vi "Curl Height.vi"(0 "Image in":T1, 1 "Coord Centre X":dbl, 2 "Coord Centre Y":dbl, 3 "Angle":dbl, 4 "Overlay Enable":bool, 5 "Measurement ROI":T8={"Left"=40.0, "Top"=75.0, "Right"=80.0, "Bottom"=3.0, "Angle"=0.0}, 6 "Measu Edge Options":T5={"Edge Polarity"=0, "Kernel Size"=5, "Width"=5, "Minimum Edge Strength"=40.0, "Interpolation Type"=enum."Zero Order", "Data Processing Method"=enum."Average"} {"Edge Polarity" items=["All Edges", "Rising Edges", "Falling Edges"]; "Minimum Edge Strength" format="%.2f"; "Width" step=2; "Kernel Size" step=2}, 7 "error in (no error)":errorcluster, 8 "Measurement Reference ROI":T8={"Left"=0.0, "Top"=0.0, "Right"=0.0, "Bottom"=280.0, "Angle"=0.0}, 9 "Measu ROI Step Size":u32=1, 10 "Measu Ref Edge Options":T5={"Edge Polarity"=0, "Kernel Size"=5, "Width"=5, "Minimum Edge Strength"=40.0, "Interpolation Type"=enum."Zero Order", "Data Processing Method"=enum."Average"} {"Edge Polarity" items=["All Edges", "Rising Edges", "Falling Edges"]; "Minimum Edge Strength" format="%.2f"; "Width" step=2; "Kernel Size" step=2}, 11 "Measu ROI Process":T7(ring)=enum."Get First + Last Edge", 12 "Measu Ref Scan Direction":u16(ring)=2 items=["Left To Right", "Right To Left", "Top To Bottom", "Bottom To Top"], 13 "Measurement ROI Scan Direction":u16(ring) items=["Left To Right", "Right To Left", "Top To Bottom", "Bottom To Top"], 14 "Calibrated Image in":T1) -> (18 "Overlay Arrows Line":T2, 20 "Curl Height":dbl format="%.2f", 21 "min value":dbl, 22 "min index(es)":i32, 23 "Curl Min Point":cluster{"X":sgl, "Y":sgl}, 27 "error out":errorcluster)   [LabVIEW 2019, in "Algorithm.lvclass"]
uses:
  FrameworkOverrides/Algorithm.lvclass
  <vilib>/vision/NI_Vision_Development_Module.lvlib
  <vilib>/vision/Image Controls.llb/IMAQ Image.ctl
  <vilib>/vision/Measure.llb/Edge Polarity.ctl
  <vilib>/vision/Measure.llb/Edge Options.ctl
panel:
  out "Image out":T1(plugin-control)
  out "Second Overlay Line":T3
  out "First Overlay Line":T4
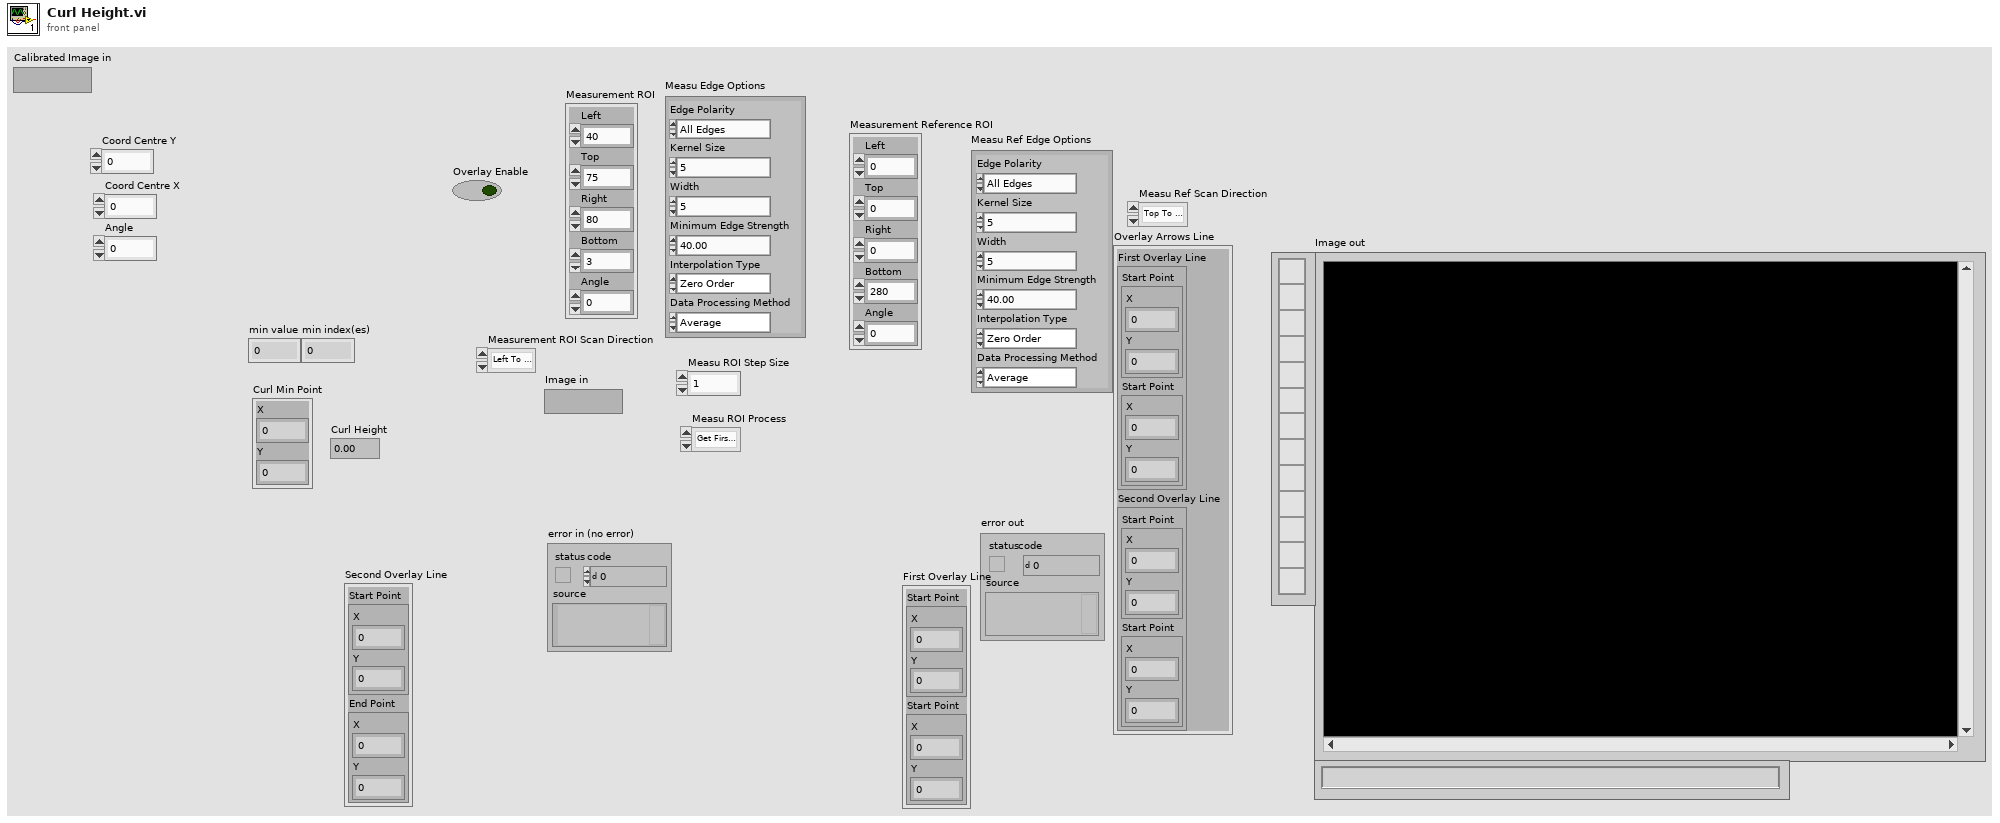
[diagram p1: front panel]
types:
  T1 = typedef "IMAQ Image.ctl" = refnum<image>
  T2 = cluster{"First Overlay Line ":cluster{"Start Point":cluster{"X":sgl, "Y":sgl}, "Start Point":cluster{"X":sgl, "Y":sgl}}, "Second Overlay Line ":cluster{"Start Point":cluster{"X":sgl, "Y":sgl}, "Start Point":cluster{"X":sgl, "Y":sgl}}}
  T3 = cluster{"Start Point":cluster{"X":sgl, "Y":sgl}, "End Point":cluster{"X":sgl, "Y":sgl}}
  T4 = cluster{"Start Point":cluster{"X":sgl, "Y":sgl}, "Start Point":cluster{"X":sgl, "Y":sgl}}
  T5 = typedef "Edge Options.ctl" = cluster{"Edge Polarity":T6, "Kernel Size":u32, "Width":u32, "Minimum Edge Strength":sgl, "Interpolation Type":enum32{"Zero Order", "Bilinear", "Quadratic", "Cubic", "Bilinear Fixed"}, "Data Processing Method":enum32{"Average", "Median"}}
  T6 = typedef "Edge Polarity.ctl" = u32
  T7 = enum16{"Get First Edge", "Get First + Last Edge", "Get All Edges", "Get Best Edge"}
  T8 = cluster{"Left":dbl, "Top":dbl, "Right":dbl, "Bottom":dbl, "Angle":dbl}
  T9 = typedef "Search Line.ctl" = cluster{"Start Point":cluster{"X":sgl, "Y":sgl}, "End Point":cluster{"X":sgl, "Y":sgl}, "Edge Info":T10[], "Edge Map":dbl[], "Calibration Valid":bool}
  T10 = typedef "Edge New.ctl" = cluster{"Location (Pixel)":cluster{"X":sgl, "Y":sgl}, "Location (Real-World)":cluster{"X":sgl, "Y":sgl}, "Distance (Pixel)":dbl, "Distance (Real-World)":dbl, "Strength":dbl, "Noise":dbl, "Rising?":bool}
  T11 = cluster{"Real World Coordinates":cluster{"X":sgl, "Y":sgl}, "Real World Coordinates":cluster{"X":sgl, "Y":sgl}}
  T12 = cluster{"Point 1":cluster{"X":sgl, "Y":sgl}, "Point 2":cluster{"X":sgl, "Y":sgl}}
  T13 = cluster{cluster{"X":sgl, sgl}, cluster{"X":sgl, "Y":sgl}}
  T14 = cluster{cluster{"X":sgl, "Y":sgl}, cluster{"X":sgl, sgl}}
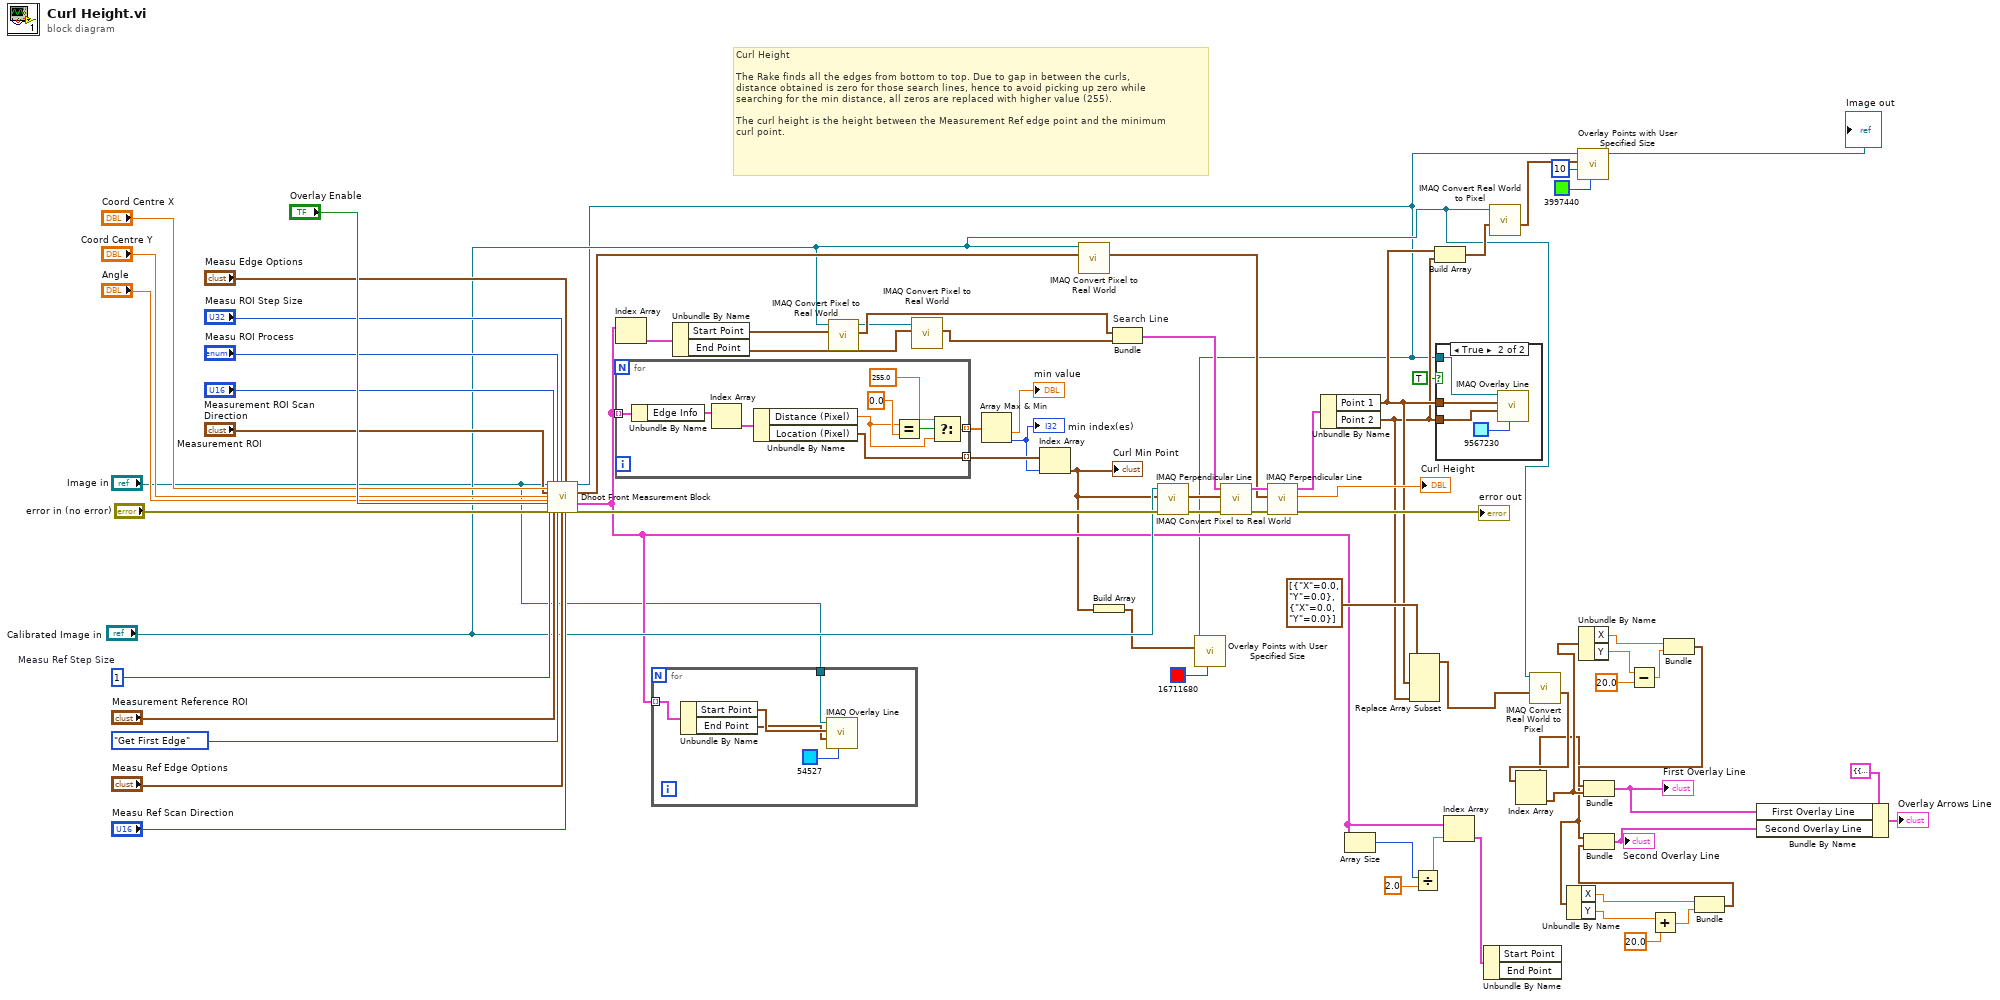
[diagram p0: block diagram]
diagram:
  w58 = u32 1  # Measu Ref Step Size
  # "Curl Height\n\nThe Rake finds all the edges from bottom to top. Due to gap in between the curls,\ndistance obtained is zero for those search lines, hence to avoid picking up zero while \nsearching for the min distance, all zeros are replaced with higher value (255).\n\nThe curl height is the height between the Measurement Ref edge point and the minimum \ncurl point."
  n1 = call "Dhoot Front Measurement Block.vi"("Image in"="Image in", "Coord Centre X"="Coord Centre X", "Measurement ROI"="Measurement ROI", "Coord Centre Y"="Coord Centre Y", "Angle"="Angle", "ROI Enable"="Overlay Enable", "Measu Ref Step Size"=w58, "error in (no error)"="error in (no error)", "Measurement ROI Scan Direction"="Measurement ROI Scan Direction", "Measurement Reference ROI"="Measurement Reference ROI", "Measu ROI Process"="Measu ROI Process", "Measu Ref Process"=T7."Get First Edge", "Measu ROI Step Size"="Measu ROI Step Size", "Measu Ref Edge Options"="Measu Ref Edge Options", "Measu Edge Options"="Measu Edge Options", "Measu Ref Scan Direction"="Measu Ref Scan Direction") -> ("Image out"=w2:T1, "Measu Ref Edge Point"=w39:cluster{"X":sgl, "Y":sgl}, "Search Lines"=w7:T9[], "error IO"=w47:errorcluster)  [unwired: 4 in, 4 out]
  "Image out" <- w2
  n2 = for {
    tunnel: w7 -> [w82] mode=indexing
    tunnel: [w75] -> w73 mode=indexing
    tunnel: [w74] -> w71 mode=indexing
    n3 = Unbundle By Name(w82) -> ("Edge Info"=w81:T10[])
    n4 = Index Array(array=w81) -> (element=w80:T10)  [unwired: 1 in]
    n5 = Unbundle By Name(w80) -> ("Distance (Pixel)"=w77:dbl, "Location (Pixel)"=w74:cluster{"X":sgl, "Y":sgl})
    n6 = Equal?(x=w77, y=0.0) -> (x = y?=w78:bool)
    n7 = Select(t=255.0, s=w78, f=w77) -> (s? t:f=w75:dbl)
  }
  n8 = Index Array(array=w7) -> (element=w69:T9)  [unwired: 1 in]
  n9 = for {
    tunnel: w7 -> [w87] mode=indexing
    tunnel: "Image in" -> [w84]
    n10 = Unbundle By Name(w87) -> ("Start Point"=w86:cluster{"X":sgl, "Y":sgl}, "End Point"=w85:cluster{"X":sgl, "Y":sgl})
    n11 = call "IMAQ Overlay Line"("Color"=u32 54527, "End Point"=w85, "Start Point"=w86, "Image"=w84) -> ()  [unwired: 6 in, 2 out]
  }
  n12 = Unbundle By Name(w69) -> ("Start Point"=w44:cluster{"X":sgl, "Y":sgl}, "End Point"=w42:cluster{"X":sgl, "Y":sgl})
  n13 = call "IMAQ Convert Pixel to Real World"("Pixel Coordinates"=w44, "Calibrated Image"="Calibrated Image in") -> ("Real World Coordinates"=w43:cluster{"X":sgl, "Y":sgl}, "Calibrated Image (duplicate)"=w40:T1)  [unwired: 4 in, 4 out]
  n14 = call "IMAQ Convert Pixel to Real World"("Pixel Coordinates"=w42, "Calibrated Image"=w40) -> ("Real World Coordinates"=w41:cluster{"X":sgl, "Y":sgl})  [unwired: 4 in, 5 out]
  n15 = Array Max & Min(array=w73) -> (min value=→"min value":dbl, min index (indices)=w70:i32)  [unwired: 2 out]
  "min index(es)" <- w70
  n16 = Index Array(array=w71, index=w70) -> (element=w4:cluster{"X":sgl, "Y":sgl})
  "Curl Min Point" <- w4
  n17 = call "IMAQ Convert Pixel to Real World"("Pixel Coordinates"=w39, "Calibrated Image"="Calibrated Image in") -> ("Real World Coordinates"=w38:cluster{"X":sgl, "Y":sgl})  [unwired: 4 in, 5 out]
  n18 = Build Array(w4) -> (w3:cluster{"X":sgl, "Y":sgl}[])
  n19 = Bundle "Search Line"("Real World Coordinates"=w43, "Real World Coordinates"=w41) -> (w68:T11)  [unwired: 1 in]
  n20 = call "IMAQ Convert Pixel to Real World"("error in (no error)"=w47, "Pixel Coordinates"=w4, "Calibrated Image"="Calibrated Image in") -> ("error out"=w46:errorcluster, "Real World Coordinates"=w45:cluster{"X":sgl, "Y":sgl})  [unwired: 3 in, 4 out]
  n21 = call "Overlay Points with User Specified Size.vi"("Color"=u32 16711680, "Points"=w3, "Image In"=w2) -> ()  [unwired: 7 in, 2 out]
  n22 = call "IMAQ Perpendicular Line"("error in (no error)"=w46, "Point"=w45, "Line"=w68) -> ("error out"=w67:errorcluster, "Perpendicular Line"=w66:T12)  [unwired: 6 in, 1 out]
  n23 = call "IMAQ Perpendicular Line"("error in (no error)"=w67, "Point"=w38, "Line"=w66) -> ("error out"=→"error out":errorcluster, "Distance"=→"Curl Height":dbl, "Perpendicular Line"=w65:T12)  [unwired: 6 in]
  n24 = Unbundle By Name(w65) -> ("Point 1"=w30:cluster{"X":sgl, "Y":sgl}, "Point 2"=w29:cluster{"X":sgl, "Y":sgl})
  n25 = Array Size(array=w7) -> (size(s)=w34:i32)
  n26 = Replace Array Subset(array=cluster{"X":sgl, "Y":sgl}[] [{"X"=0.0, "Y"=0.0}, {"X"=0.0, "Y"=0.0}] ("Point 1"), new element #1=w30, new element #2=w29) -> (w23:cluster{"X":sgl, "Y":sgl}[])  [unwired: 2 in]
  n27 = Divide(x=w34, y=2.0) -> (x/y=w33:dbl)
  n28 = Build Array(w30, w29) -> (w28:cluster{"X":sgl, "Y":sgl}[])
  n29 = case shown="True" TRUE {
    tunnel: w30 -> [_ w91]
    tunnel: w29 -> [_ w90]
    tunnel: w2 -> [_ w89]
    frame False {
    }
    frame True {
      n30 = call "IMAQ Overlay Line"("Color"=u32 9567230, "End Point"=w90, "Start Point"=w91, "Image"=w89) -> ()  [unwired: 6 in, 2 out]
    }
  }
  n31 = Index Array(array=w7, index=w33) -> (element=w37:T9)
  n32 = Unbundle By Name(w37) -> ()  [unwired: 2 out]
  n33 = call "IMAQ Convert Real World to Pixel"("Array of Real World Coordinates"=w28, "Calibrated Image"="Calibrated Image in") -> ("Array of Pixel Coordinates"=w27:cluster{"X":sgl, "Y":sgl}[])  [unwired: 4 in, 5 out]
  n34 = call "IMAQ Convert Real World to Pixel"("Array of Real World Coordinates"=w23, "Calibrated Image"="Calibrated Image in") -> ("Array of Pixel Coordinates"=w22:cluster{"X":sgl, "Y":sgl}[])  [unwired: 4 in, 5 out]
  n35 = Index Array(array=w22) -> (element #1=w13:cluster{"X":sgl, "Y":sgl}, element #2=w19:cluster{"X":sgl, "Y":sgl})  [unwired: 2 in]
  n36 = Unbundle By Name(w13) -> ("X"=w10:sgl, "Y"=w11:sgl)
  n37 = call "Overlay Points with User Specified Size.vi"("Color"=u32 3997440, "Point Diameter (5)"=u32 10, "Points"=w27, "Image In"=w2) -> ()  [unwired: 6 in, 2 out]
  n38 = Unbundle By Name(w19) -> ("X"=w18:sgl, "Y"=w17:sgl)
  n39 = Subtract(x=w17, y=sgl 20.0) -> (x-y=w15:sgl)
  n40 = Add(x=w11, y=sgl 20.0) -> (x+y=w9:sgl)
  n41 = Bundle("X"=w18, w15) -> (w14:cluster{"X":sgl, sgl})  [unwired: 1 in]
  n42 = Bundle(w14, w19) -> (w21:T13)  [unwired: 1 in]
  "First Overlay Line" <- w21
  n43 = Bundle("X"=w10, w9) -> (w8:cluster{"X":sgl, sgl})  [unwired: 1 in]
  n44 = Bundle(w13, w8) -> (w20:T14)  [unwired: 1 in]
  "Second Overlay Line" <- w20
  n45 = Bundle By Name(cluster=T2 {"First Overlay Line "={"Start Point"={"X"=0.0, "Y"=0.0}, "Start Point"={"X"=0.0, "Y"=0.0}}, "Second Overlay Line "={"Start Point"={"X"=0.0, "Y"=0.0}, "Start Point"={"X"=0.0, "Y"=0.0}}}, "First Overlay Line"=w21, "Second Overlay Line"=w20) -> (→"Overlay Arrows Line":T2)
